vi "ReadValue.vi"(3 "error in (no error)":errorcluster, 4 "Fetch/Measure":enum16{"Fetch", "Measure", ""}(ring), 5 "Measurement":T1(ring), 6 "VISA resource name":refnum<visa-resource-name>) -> (0 "error out":errorcluster, 1 "value":dbl, 2 "VISA resource name out":refnum<visa-resource-name>)   [LabVIEW 2018, in "BK Precision 983X Series.lvlib"]
uses:
  <instrlib>/BK Precision 983X Series/BK Precision 983X Series.lvlib
panel:
  out "Command":string
  # "Fetch - current reading\nMeasure - take a new reading"
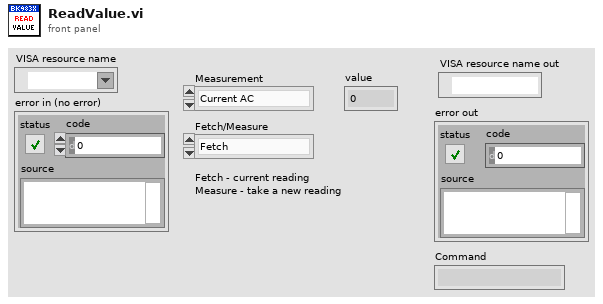
[diagram p1: front panel]
types:
  T1 = enum16{"Current AC", "Current DC", "Voltage AC", "Voltage DC", "Current Crest Factor", "Current Inrush", "Current Pos Peak", "Current Neg Peak", "Frequency", "Power Real", "Power Apparent", "Power Reactive", "Power Factor"}
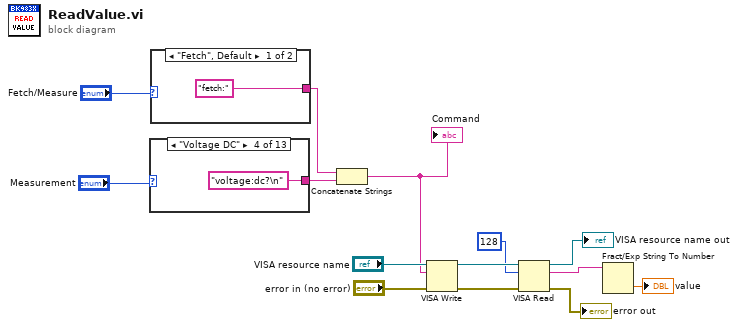
[diagram p0: block diagram]
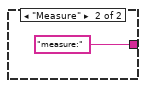
[diagram p2: hidden frame]
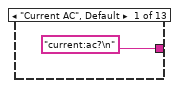
[diagram p3: hidden frame]
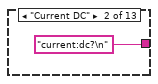
[diagram p4: hidden frame]
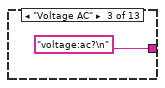
[diagram p5: hidden frame]
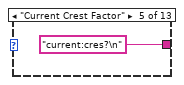
[diagram p6: hidden frame]
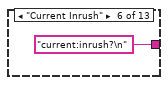
[diagram p7: hidden frame]
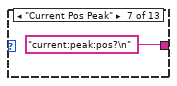
[diagram p8: hidden frame]
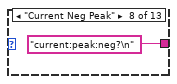
[diagram p9: hidden frame]
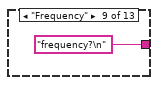
[diagram p10: hidden frame]
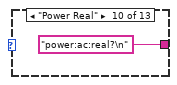
[diagram p11: hidden frame]
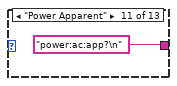
[diagram p12: hidden frame]
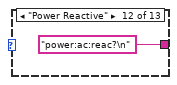
[diagram p13: hidden frame]
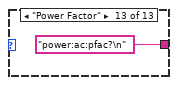
[diagram p14: hidden frame]
diagram:
  n1 = case shown="\"Voltage DC\"" "Measurement" {
    tunnel: ["current:ac?\n" "current:dc?\n" "voltage:ac?\n" "voltage:dc?\n" "current:cres?\n" "current:inrush?\n" "current:peak:pos?\n" "current:peak:neg?\n" "frequency?\n" "power:ac:real?\n" "power:ac:app?\n" "power:ac:reac?\n" "power:ac:pfac?\n"] -> w4
    frame "Current AC", Default {
    }
    frame "Current DC" {
    }
    frame "Voltage AC" {
    }
    frame "Voltage DC" {
    }
    frame "Current Crest Factor" {
    }
    frame "Current Inrush" {
    }
    frame "Current Pos Peak" {
    }
    frame "Current Neg Peak" {
    }
    frame "Frequency" {
    }
    frame "Power Real" {
    }
    frame "Power Apparent" {
    }
    frame "Power Reactive" {
    }
    frame "Power Factor" {
    }
  }
  n2 = case shown="\"Fetch\", Default" "Fetch/Measure" {
    tunnel: ["fetch:" "measure:"] -> w1
    frame "Fetch", Default {
    }
    frame "Measure" {
    }
  }
  n3 = Concatenate Strings(w1, w4) -> (w5:string)
  "Command" <- w5
  n4 = VISA Write(VISA resource name="VISA resource name", write buffer=w5, error in (no error)="error in (no error)") -> (VISA resource name out=w14:refnum<visa-resource-name>, error out=w13:errorcluster)  [unwired: 1 out]
  n5 = VISA Read(VISA resource name=w14, byte count=u32 128, error in (no error)=w13) -> (VISA resource name out=→"VISA resource name out":refnum<visa-resource-name>, read buffer=w12:string, error out=→"error out":errorcluster)  [unwired: 1 out]
  n6 = Fract/Exp String To Number(string=w12) -> (number=→"value":dbl)  [unwired: 3 in, 1 out]
